vi "Get Input Parameter.vi"(8 "error in (no error)":errorcluster, 10 "Control Name":string, 11 "VI Call In":refnum<class "VI Call.lvclass">) -> (0 "error out":errorcluster, 2 "Value":variant)   [LabVIEW 2020, in "VI Call.lvclass"]
uses:
  VI Call.lvclass
  VI Call.lvclass/VI Call.ctl
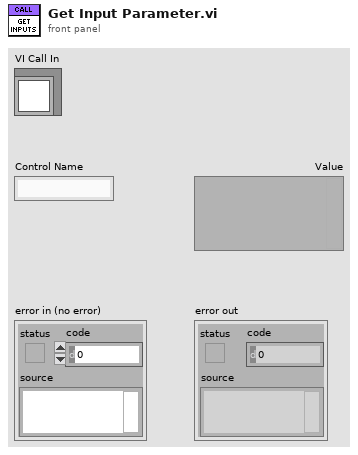
[diagram p1: front panel]
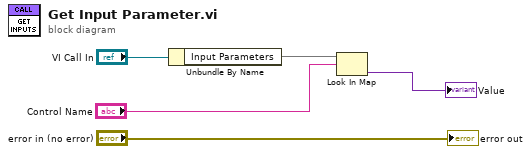
[diagram p0: block diagram]
diagram:
  n1 = Unbundle By Name("VI Call In") -> ("Input Parameters"=w3:map{string, variant})
  n2 = Look In Map(map=w3, key="Control Name") -> (value=→"Value":variant)  [unwired: 1 in, 1 out]
  "error out" <- "error in (no error)"
